vi "TCPIP H.vi"(0 "产品ID+X 2":string, 1 "LOT NO.":string, 2 "架子ID":string, 3 "托盘ID+1":string, 4 "TESTRLT":string, 5 "MES字符串":string, 6 "作业员ID":string, 7 "基板箱ID+时间日期":string, 8 "机器名称":string, 9 "error in (no error)":errorcluster caption="错误输入（无错误）", 10 "线别":string, 11 "抓图？":bool, 13 "path to JPEG file":path caption="JPEG文件路径") -> (12 "x = y?":bool, 14 "Y&N":string, 15 "系统消息":string, 16 "体部":string, 17 "头部":string, 19 "error out":errorcluster caption="错误输出")   [LabVIEW 2014]
panel:
  out "RESULT":cluster{"Result":bool, "Message":string}
  in  "STATE":T1(ring)=enum."RLT_PASS"
  in  "TCP超时":u64=3000
  in  "SFC":string
  # "http://10.9.30.175:50100\n/manufacturing/IntegrationServlet?InterType=XML&message=\n ERROR<PRODUCTION_REQUEST><NC_LOG_COMPLETE><SITE>A157</SITE><OWNER TYPE=\"USER\">TEST</OWNER><NC_CONTEXT>\n0105442MF01140002</NC_CONTEXT><QTY></QTY><IDENTIFIER></IDENTIFIER><FAILURE_ID></FAILURE_ID><DEFECT_COUNT>1</DEFECT_COUNT>\n<COMMENTS></COMMENTS><DATE_TIME></DATE_TIME><RESOURCE>A-6-Z-TEST</RESOURCE><OPERATION>Z-TEST</OPERATION><ROOT_CAUSE_OPER>\n</ROOT_CAUSE_OPER><NC_CODE>Z-TEST_FAIL</NC_CODE><ACTIVITY>XML</ACTIVITY></NC_LOG_COMPLETE></PRODUCTION_REQUEST>\n!erpautogy03!1234567@byd!ERROR,11V1.0,11V1.0!"
  # "[BYD_MES]\nSITE=X157\nOPERATION=Z-CS\nRESOURCE=Z-QT-01-F3-YQ-BLSJQCS-01\nNC_CODE=Z-CS_FAIL\nIP=10.3.3.114\nPORT=50000\nURL=/manufacturing/IntegrationServlet?InterType=XML&message="
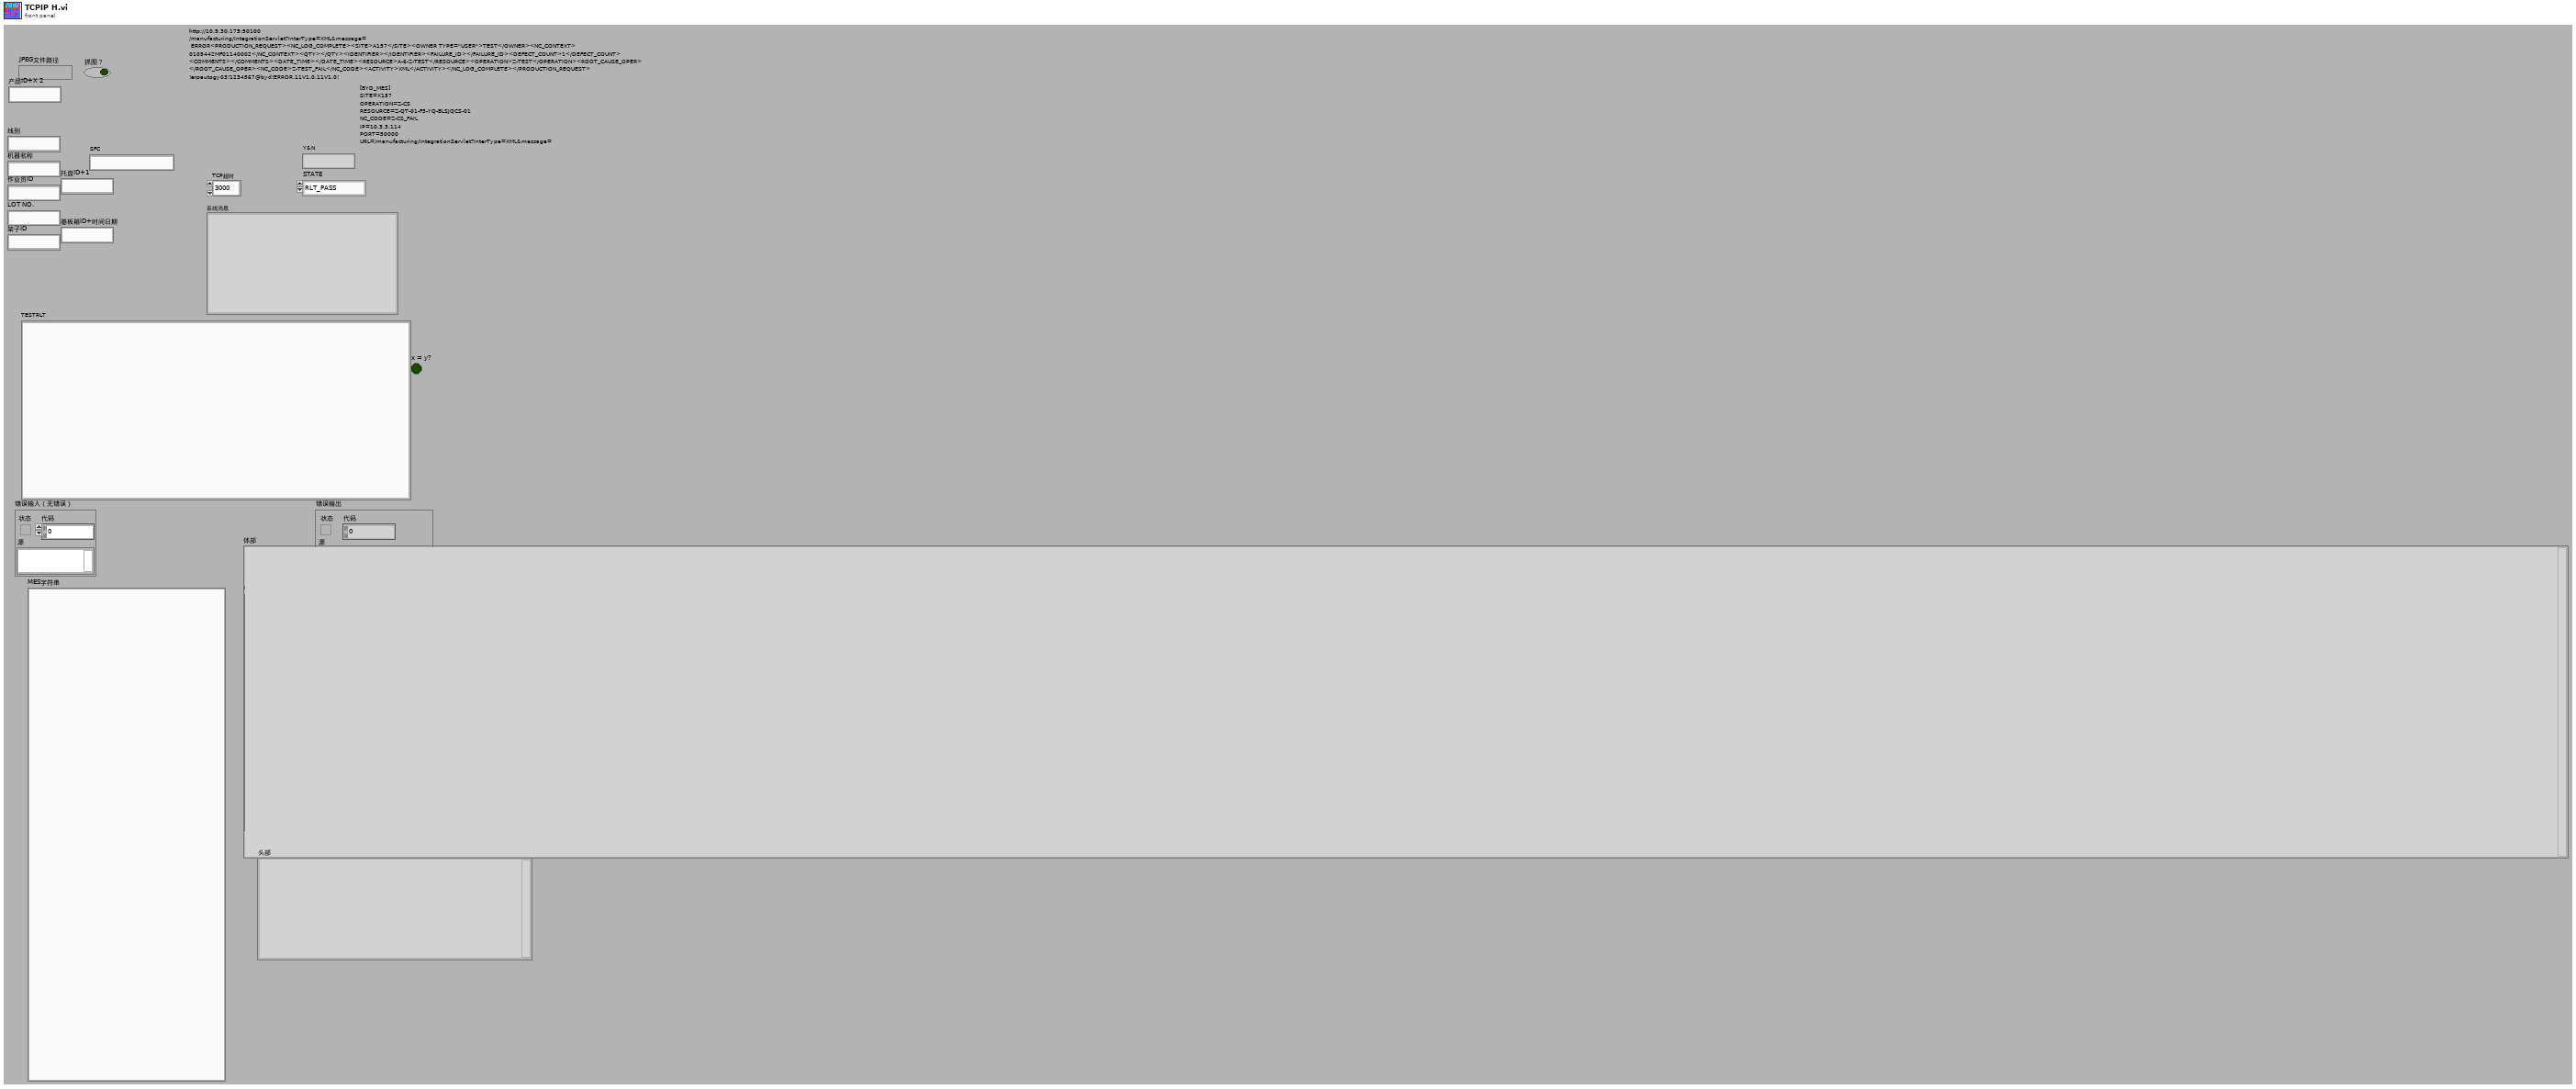
[diagram p1: front panel]
types:
  T1 = enum16{"USER_CHECK", "SFC_CHECK", "RLT_PASS", "RLT_ERROR", "RES_AREA"}
  T2 = cluster{"线别":string, "机器名称":string, "作业员ID":string, "LOT NO.":string, "架子ID":string, "托盘ID+1":string, "产品ID+X":string, "基板箱ID+时间日期":string}
  T3 = typedef "imagedata.ctl" = cluster{"image type":i32, "image depth":i32, "image":u8[], "mask":u8[], "colors":u32[], "Rectangle":cluster{"left":i16, "top":i16, "right":i16, "bottom":i16}}
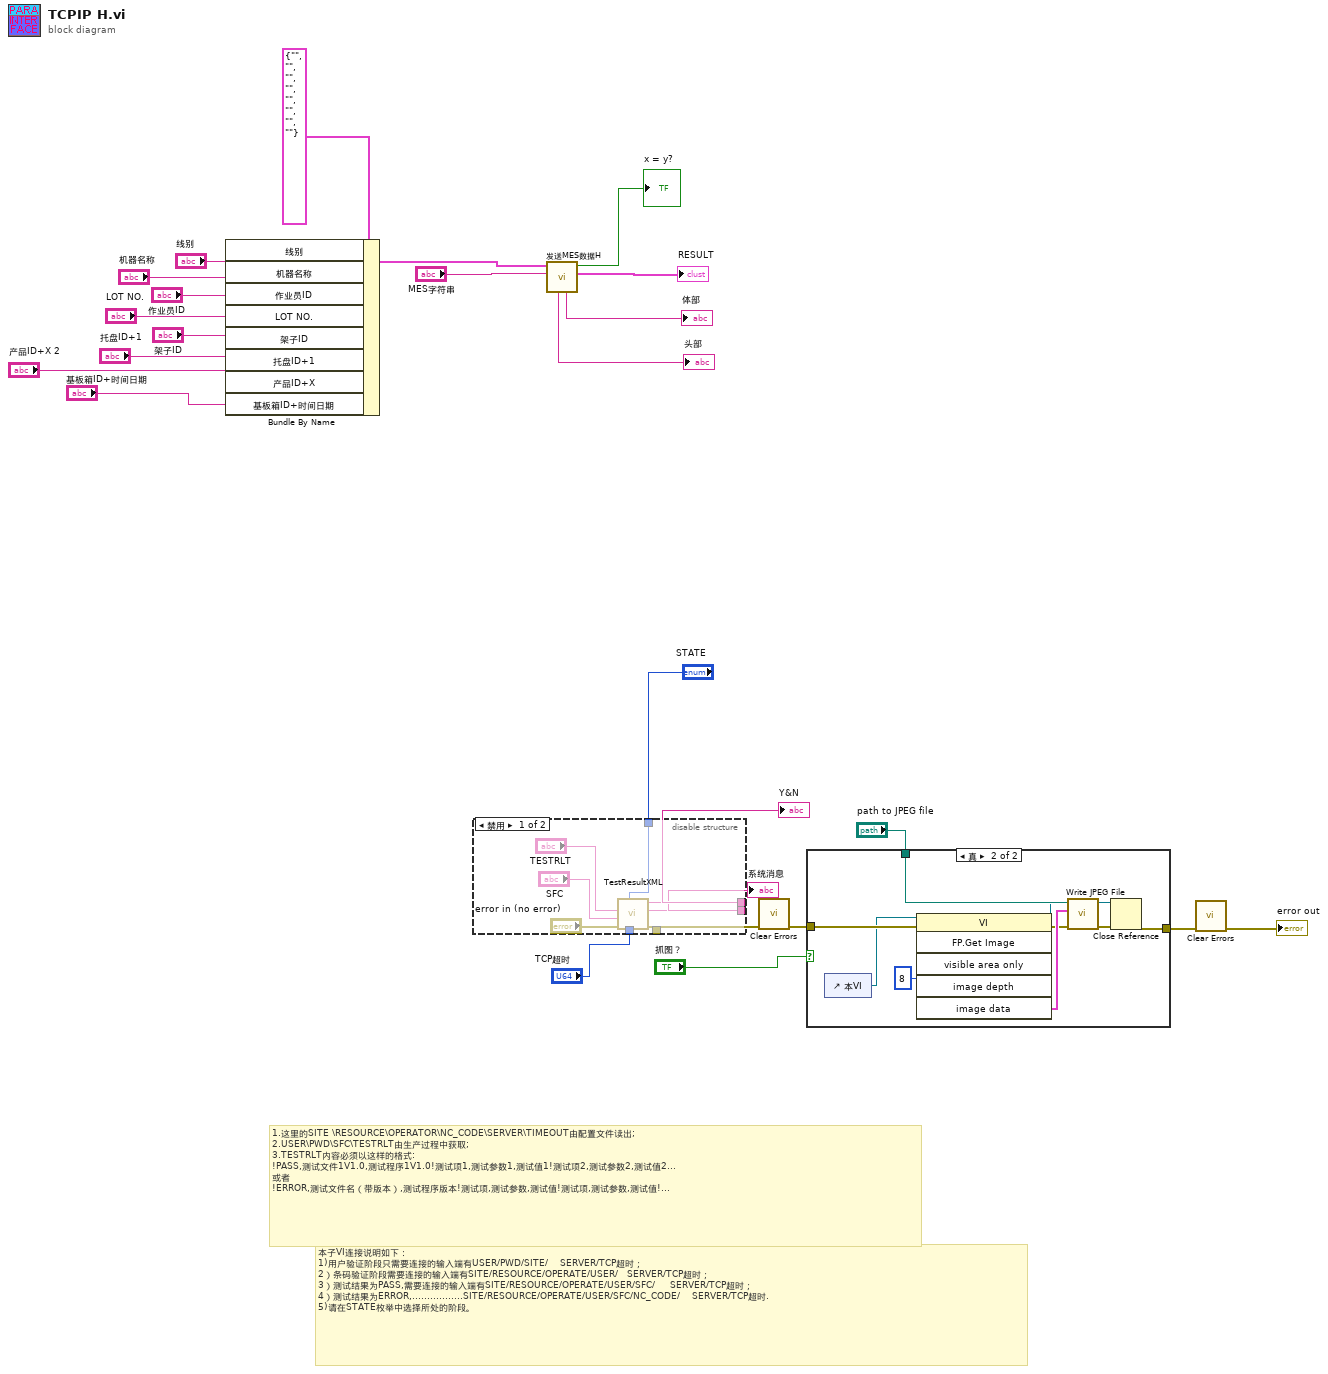
[diagram p0: block diagram]
diagram:
  # "本子VI连接说明如下：\n1)用户验证阶段只需要连接的输入端有USER/PWD/SITE/    SERVER/TCP超时；\n2）条码验证阶段需要连接的输入端有SITE/RESOURCE/OPERATE/USER/   SERVER/TCP超时；\n3）测试结果为PASS,需要连接的输入端有SITE/RESOURCE/OPERATE/USER/SFC/     SERVER/TCP超时；\n4）测试结果为ERROR,.................SITE/RESOURCE/OPERATE/USER/SFC/NC_CODE/    SERVER/TCP超时.\n5)请在STATE枚举中选择所处的阶段。"
  # "1.这里的SITE \\RESOURCE\\OPERATOR\\NC_CODE\\SERVER\\TIMEOUT由配置文件读出;\n2.USER\\PWD\\SFC\\TESTRLT由生产过程中获取;\n3.TESTRLT内容必须以这样的格式:\n!PASS,测试文件1V1.0,测试程序1V1.0!测试项1,测试参数1,测试值1!测试项2,测试参数2,测试值2...\n或者\n!ERROR,测试文件名（带版本）,测试程序版本!测试项,测试参数,测试值!测试项,测试参数,测试值!..."
  n1 = Bundle By Name(cluster=T2 {"线别"="", "机器名称"="", "作业员ID"="", "LOT NO."="", "架子ID"="", "托盘ID+1"="", "产品ID+X"="", "基板箱ID+时间日期"=""} ("MES配置"), "线别"="线别", "机器名称"="机器名称", "作业员ID"="作业员ID", "LOT NO."="LOT NO.", "架子ID"="架子ID", "托盘ID+1"="托盘ID+1", "产品ID+X"="产品ID+X 2", "基板箱ID+时间日期"="基板箱ID+时间日期") -> (w2:T2)
  n2 = disable-structure shown="禁用" {
    disable-tunnel: "TCP超时" -> [w32 _]
    disable-tunnel: [w31 _] -> w20
    disable-tunnel: [w30 _] -> w19
    disable-tunnel: [w27 _] -> w18
    disable-tunnel: "STATE" -> [w26 _]
    frame Disabled {
      n3 = call "TestResultXML.vi"("TCP超时"=w32, "STATE"=w26, "error in (no error)"="error in (no error)", "SFC"="SFC", "TESTRLT"="TESTRLT") -> ("error out"=w27:errorcluster, "SYSTEM INFO"=w30:string, "Y&N"=w31:string)  [unwired: 2 in]
    }
    frame Enabled {
    }
  }
  "Y&N" <- w20
  "系统消息" <- w19
  n4 = call "发送MES数据H.vi"("Data(IN)"="MES字符串", "MES配置"=w2) -> ("RESULT"=→"RESULT":cluster{"Result":bool, "Message":string}, "x = y?"=→"x = y?":bool, "body 2"=→"体部":string, "headers"=→"头部":string)  [unwired: 6 in]
  n5 = call <vilib>:"Clear Errors.vi"("error in (no error)"=w18) -> ("error out"=w13:errorcluster)  [unwired: 5 in, 1 out]
  n6 = case shown="真" "抓图？" {
    tunnel: w13 -> [w34 w43]
    tunnel: "path to JPEG file" -> [_ w38]
    tunnel: [w34 w35] -> w16
    frame False {
    }
    frame True {
      n7 = control-ref of="本VI"() -> (w42:refnum<vi>)
      n8 = invoke class="VI" method="FP.Get Image"(reference=w42, error in=w43, "image depth"=8 ("图像深度")) -> (reference out=w36:refnum<vi>, error out=w39:errorcluster, "image data"=w40:T3)  [unwired: 3 in, 3 out]
      n9 = call <vilib>:"Write JPEG File.vi"("error in (no error)"=w39, "image data"=w40, "path to JPEG file"=w38) -> ("error out"=w37:errorcluster)  [unwired: 7 in, 1 out]
      n10 = Close Reference(reference=w36, error in (no error)=w37) -> (error out=w35:errorcluster)
    }
  }
  n11 = call <vilib>:"Clear Errors.vi"("error in (no error)"=w16) -> ("error out"=→"error out":errorcluster)  [unwired: 5 in, 1 out]
